vi "Sonar Strafe.vi"(6 "reinitialize? (F)":bool=TRUE, 8 "Sonar Side":string="Sonar Left Side", 9 "Desired Wall Distance":dbl=32.0) -> (0 "Distance Reached?":bool=TRUE, 1 "Joy Y":dbl, 3 "Joy X":dbl)   [LabVIEW 2014]
uses:
  <vilib>/Rock Robotics/WPI/Ultrasonic/WPI_SonarMB1010AnalogRefNum Registry Get.vi
  <vilib>/Rock Robotics/WPI/Ultrasonic/WPI_SonarMB1010AnalogGetRange.vi
  <vilib>/addons/control/pid/pid.llb/PID (DBL).vi
  <vilib>/addons/control/pid/NI_PID_pid.lvlib
panel:
  in  "Forward Output Range":cluster{"output high":dbl, "output low":dbl}={"output high"=0.75, "output low"=-0.75} {"output low" format="%.2f"; "output high" format="%.2f"}
  in  "Forward PID gains":T1={"proportional gain (Kc)"=0.1, "integral time (Ti, min)"=1.0, "derivative time (Td, min)"=0.0} {"derivative time (Td, min)" format="%.3f"; "integral time (Ti, min)" format="%.3f"; "proportional gain (Kc)" format="%.3f"}
  in  "Forward Range":dbl=0.8
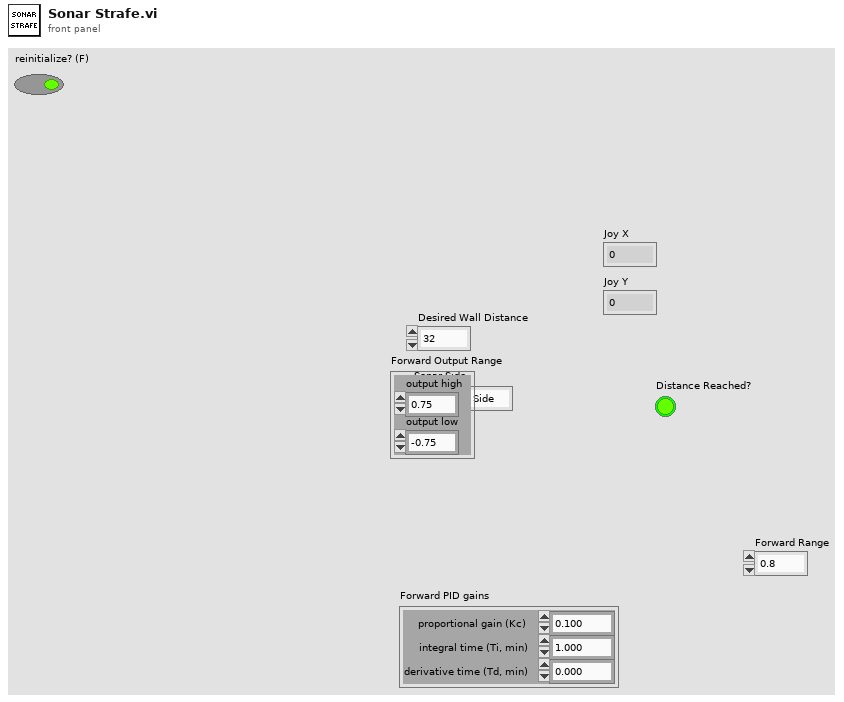
[diagram p1: front panel]
types:
  T1 = cluster{"proportional gain (Kc)":dbl, "integral time (Ti, min)":dbl, "derivative time (Td, min)":dbl}
  T2 = typedef "WPI_SonarMB1010AnalogDeviceRef.ctl" = cluster{"AIDeviceRef":T3, "Scaling factor (V/in)":dbl, "Average Bits":u8}
  T3 = typedef "WPI_AnalogChannelDevRef.ctl" = cluster{"DevStatus":errorcluster, "Controller":T4, "Analog Channel":T5}
  T4 = typedef "FPGA_TypedefAnalogModule.ctl" = enum16{"Controller 1"}
  T5 = typedef "FPGA_AIChannel.ctl" = enum8{"AI 0", "AI 1", "AI 2", "AI 3", "AI MXP 0", "AI MXP 1", "AI MXP 2", "AI MXP 3", "Invalid"}
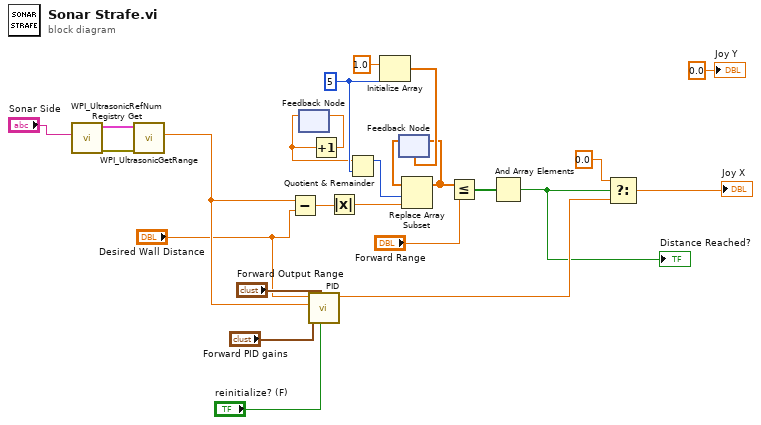
[diagram p0: block diagram]
diagram:
  w6 = 5 ("dimension size")
  n1 = call-poly <vilib>:"WPI_UltrasonicRefNum Registry Get.vi"("refnum name"="Sonar Side") -> ("error out"=w24:errorcluster, "SonarMB1010AnalogDevRef"=w25:T2)  [unwired: 9 in]
  n2 = call-poly <vilib>:"WPI_UltrasonicGetRange.vi"("error in"=w24, "SonarMB1010AnalogDevRef"=w25) -> ("Distance"=w16:dbl)  [unwired: 7 in, 2 out]
  n3 = Subtract(x=w16, y="Desired Wall Distance") -> (x-y=w21:dbl)
  n4 = feedback #1() -> (w4:dbl)  [unwired: 1 in]
  n5 = call-poly <vilib>:"PID.vi"("reinitialize? (F)"="reinitialize? (F)", "output range"="Forward Output Range", "PID gains"="Forward PID gains", "process variable"=w16, "setpoint"="Desired Wall Distance") -> ("output"=w12:dbl)  [unwired: 5 in, 1 out]
  n6 = Increment(x=w4) -> (x+1=w7:dbl)
  n7 = feedback-in #1(w7) -> ()
  n8 = Absolute Value(x=w21) -> (abs(x)=w8:dbl)
  n9 = Quotient & Remainder(x=w4, y=w6) -> (x-y*floor(x/y)=w5:i32)  [unwired: 1 out]
  n10 = Initialize Array(1.0 ("element"), w6) -> (w10:dbl[])
  n11 = feedback #2(w10) -> (w9:dbl[])
  n12 = Replace Array Subset(array=w9, new element=w8, index=w5) -> (w3:dbl[])
  n13 = feedback-in #2(w3) -> ()
  n14 = Less Or Equal?(x=w3, y="Forward Range") -> (x <= y?=w2:bool[])
  n15 = And Array Elements(Boolean array=w2) -> (logical AND=w1:bool)
  "Distance Reached?" <- w1
  n16 = Select(t=0.0, s=w1, f=w12) -> (s? t:f=→"Joy X":dbl)
  "Joy Y" <- 0.0 ("Joy Y")
